vi "CRYProject Editor PART TS Save.vi"(11 "pSaveName":path) -> ()   [LabVIEW 2013]
uses:
  CRYProject Editor Global.vi
  CRYMainGlobal.vi
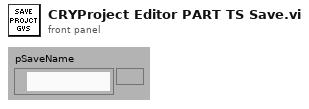
[diagram p1: front panel]
types:
  T1 = typedef "CRYTS.ctl" = cluster{"No.TS":u16, "TS File Path":path, "TS Name":string, "EditStepName":string, "Steps":T2[], "New State":bool, "Change State":bool, "Flattened CurveLib Data":string, "Document Data":string, "EditStepNo":u16, "Operator Start File":string, "Sequence Type":string, "Sequence Language":string}
  T2 = typedef "CRYStep.ctl" = cluster{"No.VI":i32, "Category":string, "StepName":string, "Seq setup flattened":string, "Comment":string, "Steps config.":bool[], "Jump config":i32[], "Start":dbl, "Increment":dbl, "Name":string, "Unit":string, "Y data":u16, "Y prefix":string, "Y dB ref":dbl, "Y unit":string, "Repeat State Array":cluster{"Start":dbl, "Increment":dbl, "Count":i32, "Num":i32}[]}
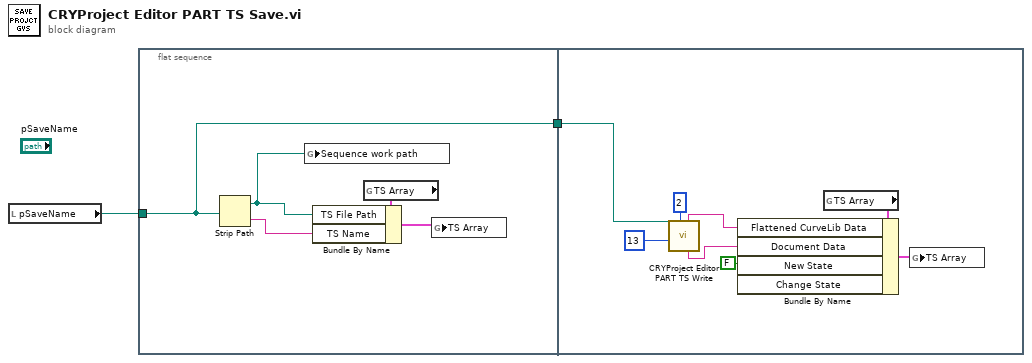
[diagram p0: block diagram]
diagram:
  n1 = local read "pSaveName"() -> (w1:path)
  n2 = flat-sequence {
    tunnel: w1 -> [w7]
    tunnel: [w7] -> w2
    tunnel: w2 -> [w11]
    frame #0 {
      n3 = Strip Path(path=w7) -> (stripped path=w4:path, name=w3:string)
      n4 = global write "CRYMainGlobal.vi" "Sequence work path"(w4) -> ()
      n5 = global read "CRYProject Editor Global.vi" "TS Array"() -> (w6:T1)
      n6 = Bundle By Name(cluster=w6, "TS File Path"=w4, "TS Name"=w3) -> (w5:T1)
      n7 = global write "CRYProject Editor Global.vi" "TS Array"(w5) -> ()
    }
    frame #1 {
      w10 = FALSE ("New State")
      n8 = call "CRYProject Editor PART TS Write.vi"("Channels"=2, "Version"=u16 13, "pSaveName"=w11) -> ("Flatten Doc Data"=w13:string, "Flatten Curve Data"=w9:string)  [unwired: 3 in, 4 out]
      n9 = global read "CRYProject Editor Global.vi" "TS Array"() -> (w15:T1)
      n10 = Bundle By Name(cluster=w15, "Flattened CurveLib Data"=w9, "Document Data"=w13, "New State"=w10, "Change State"=w10) -> (w12:T1)
      n11 = global write "CRYProject Editor Global.vi" "TS Array"(w12) -> ()
    }
  }
